vi "List Phone Numbers Recursive.vi"(8 "error in (no error)":errorcluster, 10 "nextToken":string, 11 "Phone Number":refnum<class "Phone Number.lvclass">) -> (0 "error out":errorcluster, 3 "Phone Numbers Opted Out":refnum<class "Phone Number.lvclass">[](array[class]))   [LabVIEW 2015, in "NI_AWS_SNS.lvlib" / "Phone Number.lvclass"]
uses:
  Phone Number.lvclass
  Core/HTTP Request/Request Options.ctl
  Core/HTTP Request/Name Value Pair.ctl
  Phone Number.lvclass/Phone Number.ctl
  Write Phone Number.vi
  Core/HTTP Request/HTTP Request.lvclass
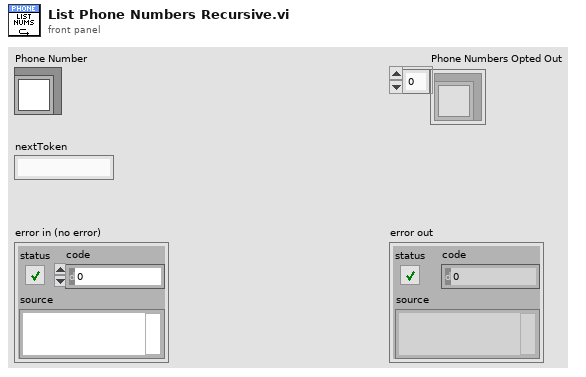
[diagram p1: front panel]
types:
  T1 = typedef "NI_AWS_Core.lvlib/HTTP Request.lvclass/Name Value Pair.ctl" = cluster{"name":string, "value":string}
  T2 = typedef "NI_AWS_Core.lvlib/HTTP Request.lvclass/Request Options.ctl" = cluster{"request headers":T1[], "request parameters":T1[], "request body":string}
  T3 = typedef "NI_AWS_Core.lvlib/HTTP Request.lvclass/Response.ctl" = cluster{"Headers":string, "Body":string}
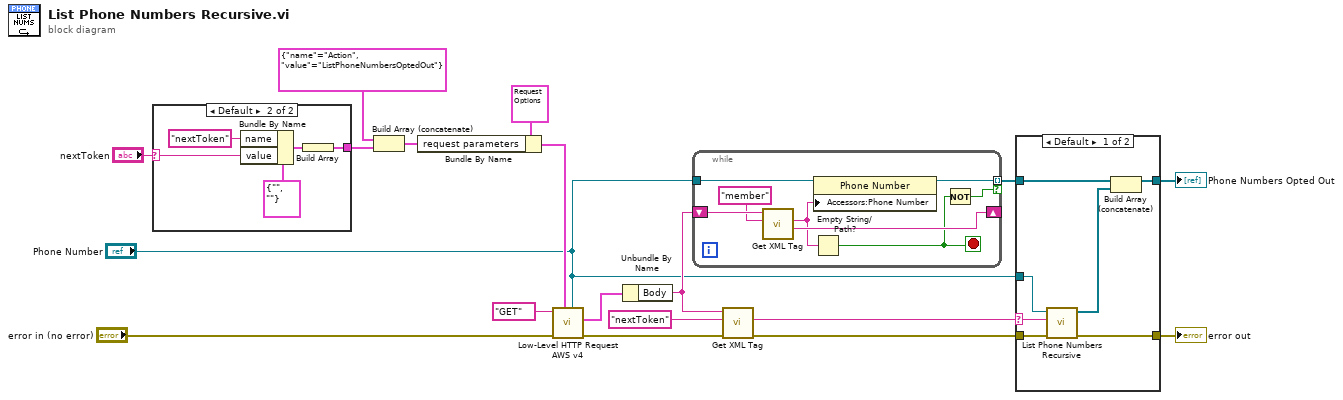
[diagram p0: block diagram]
diagram:
  n1 = case shown="Default" "nextToken" {
    selector: "nextToken" -> [_ w23]
    tunnel: [_ w19] -> w16
    frame "" {
    }
    frame Default {
      n2 = Bundle By Name(cluster=T1 {"name"="", "value"=""} ("Name Value Pair"), "name"="nextToken", "value"=w23) -> (w21:T1)
      n3 = Build Array(w21) -> (w19:T1[])
    }
  }
  n4 = Build Array (concatenate)(T1 {"name"="Action", "value"="ListPhoneNumbersOptedOut"} ("Name Value Pair"), w16) -> (w14:T1[])
  n5 = Bundle By Name(cluster=T2 {"request headers"=[], "request parameters"=[{"name"="Action", "value"="ListQueues"}], "request body"=""} ("Request Options"), "request parameters"=w14) -> (w13:T2)
  n6 = call "Low-Level HTTP Request AWS v4.vi"("AWS Core"="Phone Number", "Request Options"=w13, "error in (no error)"="error in (no error)", "HTTP-Verb"="GET") -> ("error out"=w3:errorcluster, "Response"=w18:T3)  [unwired: 5 in, 1 out]
  n7 = Unbundle By Name(w18) -> ("Body"=w9:string)
  n8 = while {
    shift-right: [w29] -> _
    shift-left: w9 -> [w31]
    tunnel: "Phone Number" -> [w28]
    tunnel: [w27] -> w6 mode=indexing if=w25
    stop <- w24 stop-if-true
    n9 = call "Get XML Tag.vi"("Tag name"="member", "XML String in"=w31) -> ("Remaining string"=w29:string, "Tag value"=w26:string)  [unwired: 5 in, 3 out]
    n10 = Empty String/Path?(string/path=w26) -> (empty?=w24:bool)
    n11 = property class="Phone Number"(reference=w28, "Accessors:Phone Number"=w26) -> (reference out=w27:refnum<class "Phone Number.lvclass">)  [unwired: 1 in, 1 out]
    n12 = Not(x=w24) -> (.not. x?=w25:bool)
  }
  n13 = call "Get XML Tag.vi"("error in (no error)"=w3, "Tag name"="nextToken", "XML String in"=w9) -> ("error out"=w2:errorcluster, "Tag value"=w7:string)  [unwired: 4 in, 3 out]
  n14 = case shown="Default" w7 {
    selector: w7 -> [w37 _]
    tunnel: w6 -> [w36 w40]
    tunnel: [w35 w40] -> w5
    tunnel: w2 -> [w38 w39]
    tunnel: [w34 w39] -> w4
    tunnel: "Phone Number" -> [w32 _]
    frame Default {
      n15 = call "List Phone Numbers Recursive.vi"("error in (no error)"=w38, "nextToken"=w37, "Phone Number"=w32) -> ("error out"=w34:errorcluster, "Phone Numbers Opted Out"=w33:refnum<class "Phone Number.lvclass">[])  [unwired: 7 in]
      n16 = Build Array (concatenate)(w36, w33) -> (w35:refnum<class "Phone Number.lvclass">[])
    }
    frame "" {
    }
  }
  "error out" <- w4
  "Phone Numbers Opted Out" <- w5
